vi "Actor Destroy.vi"(11 "Dev Actor in":refnum<class "Dev Actor.lvclass">) -> (3 "Dev Actor out":refnum<class "Dev Actor.lvclass">)   [LabVIEW 2021, in "Dev Actor.lvlib" / "Dev Actor.lvclass"]
uses:
  Dev Actor.lvclass
  <vilib>/jettl/jettl/jettl/Msg Strategy/Msg Strategy.lvclass
  Dev Actor.lvclass/Dev Actor.ctl
  <vilib>/jettl/jettl/jettl/Actor/Actor.lvclass
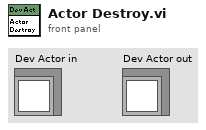
[diagram p1: front panel]
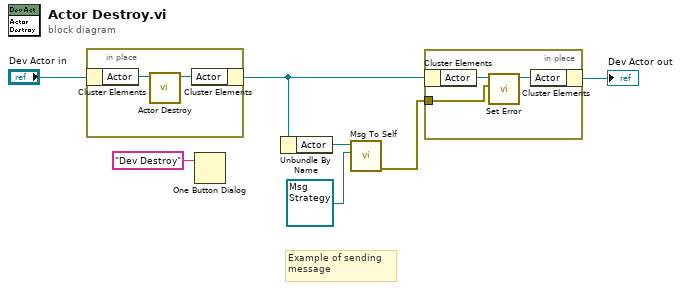
[diagram p0: block diagram]
diagram:
  # "Example of sending message"
  n1 = in-place {
    n2 = in-place-cluster #1("Dev Actor in") -> ("Actor"=w9:refnum<class "Actor.lvclass">)
    n3 = call-dynamic "Actor Destroy.vi"("Actor Destroy in"=w9) -> ("Actor Destroy out"=w8:refnum<class "Actor.lvclass">)  [unwired: 10 in]
    n4 = in-place-cluster #1("Actor"=w8) -> (w2:refnum<class "Dev Actor.lvclass">)
  }
  n5 = One Button Dialog(message="Dev Destroy") -> ()  [unwired: 1 in, 1 out]
  n6 = Unbundle By Name(w2) -> ("Actor"=w6:refnum<class "Actor.lvclass">)
  n7 = call-dynamic "Msg To Self.vi"("Msg"=refnum<class "Msg Strategy.lvclass"> refnum, "Actor in"=w6) -> ("error out"=w1:errorcluster)  [unwired: 9 in]
  n8 = in-place {
    in-place-border: w1 -> [w10]
    n9 = in-place-cluster #2(w2) -> ("Actor"=w12:refnum<class "Actor.lvclass">)
    n10 = call-dynamic "Set Error.vi"("Error"=w10, "Actor in"=w12) -> ("Actor out"=w11:refnum<class "Actor.lvclass">)  [unwired: 9 in]
    n11 = in-place-cluster #2("Actor"=w11) -> (→"Dev Actor out":refnum<class "Dev Actor.lvclass">)
  }
